vi "Simulacion_Planta_control_tustin.vi"() -> ()   [LabVIEW 2012]
panel:
  in  "stop":bool
  in  "valor deseado":dbl=700.0
  in  "u_ini":dbl
  in  "error_ini":dbl
  in  "Y(k-2)":dbl
  in  "Y(k-1)":dbl
  out "Waveform Chart":dbl(graph)=699.9999999999991
  in  "T":dbl=0.001
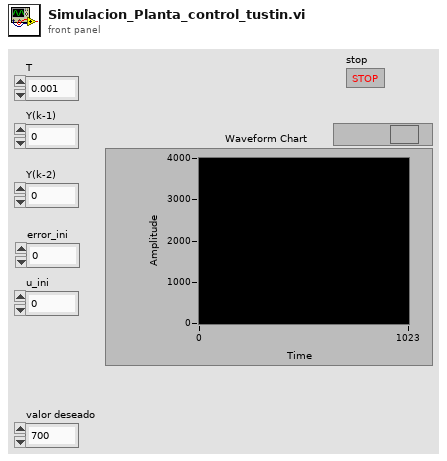
[diagram p1: front panel]
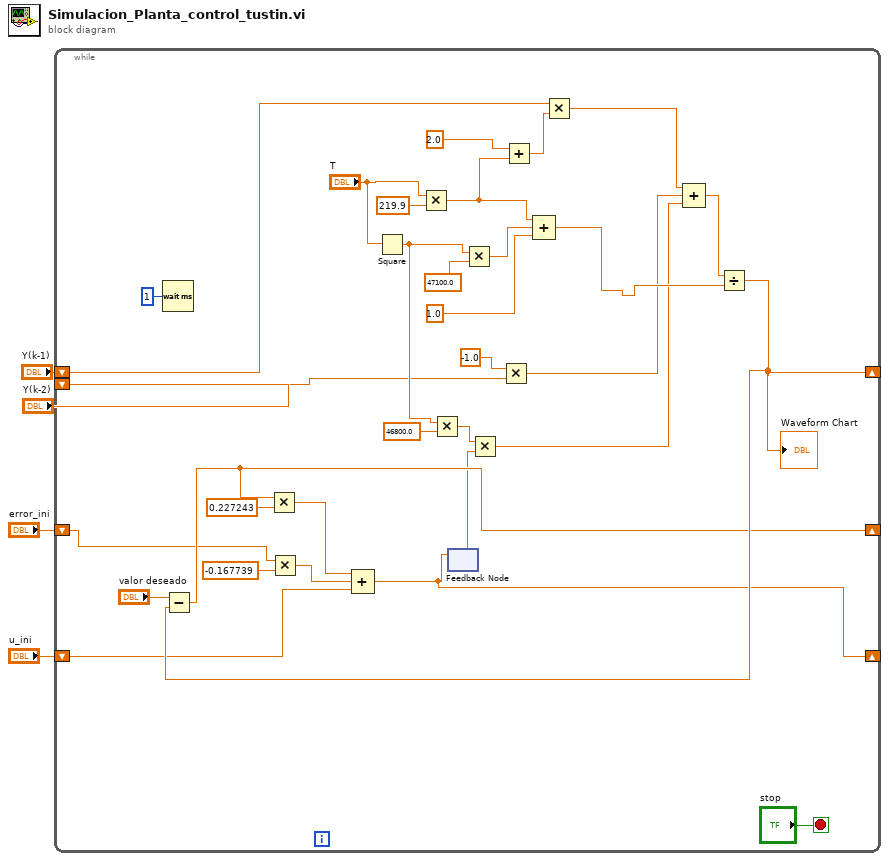
[diagram p0: block diagram]
diagram:
  n1 = while {
    shift-right: [w17] -> _
    shift-left: "Y(k-1)" -> [w29]
    shift-left: "Y(k-2)" -> [w21]
    shift-right: [w12] -> _
    shift-left: "error_ini" -> [w11]
    shift-right: [w9] -> _
    shift-left: "u_ini" -> [w8]
    stop <- "stop" stop-if-true
    n2 = Wait (ms)(milliseconds to wait=u32 1) -> ()  [unwired: 1 out]
    n3 = Multiply(x=w11, y=-0.167739) -> (x*y=w16:dbl)
    n4 = Square(x="T") -> (x^2=w25:dbl)
    n5 = Multiply(x="T", y=219.9) -> (x*y=w31:dbl)
    n6 = Multiply(x=w25, y=46800.0) -> (x*y=w24:dbl)
    n7 = feedback #1() -> (w10:dbl)  [unwired: 1 in]
    n8 = Multiply(x=w25, y=47100.0) -> (x*y=w34:dbl)
    n9 = Multiply(x=w24, y=w10) -> (x*y=w22:dbl)
    n10 = Multiply(x=-1.0, y=w21) -> (x*y=w20:dbl)
    n11 = Add(x=2.0, y=w31) -> (x+y=w30:dbl)
    n12 = Compound Arithmetic op=ADD(w31, w34, 1.0 ("value")) -> (w23:dbl)
    n13 = Multiply(x=w29, y=w30) -> (x*y=w28:dbl)
    n14 = Compound Arithmetic op=ADD(w28, w20, w22) -> (w27:dbl)
    n15 = Divide(x=w27, y=w23) -> (x/y=w17:dbl)
    "Waveform Chart" <- w17
    n16 = Subtract(x="valor deseado", y=w17) -> (x-y=w12:dbl)
    n17 = Multiply(x=w12, y=0.227243) -> (x*y=w15:dbl)
    n18 = Compound Arithmetic op=ADD(w15, w16, w8) -> (w9:dbl)
    n19 = feedback-in #1(w9) -> ()
  }
